vi "DIO 8-bit Bank.vi"(1 "DIO 7:0 Refnum":refnum<k21>, 2 "OUT 7:0":u8 format="%08b", 3 "DIR 7:0":u8 format="%08b") -> (0 "IN 7:0":u8 format="%08d")   [LabVIEW 2013]
uses:
  <vilib>/rvi/eio/common/nirviEmuTemplateMethod_errors.vi
  <vilib>/eio/EIOMethodNode/EIOMethodNode.xnode
  <vilib>/eio/EIONode/EIONode.xnode
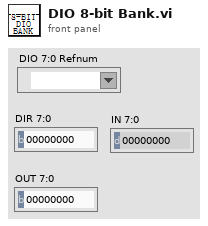
[diagram p1: front panel]
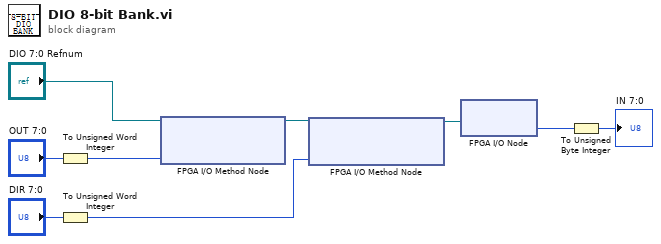
[diagram p0: block diagram]
diagram:
  n1 = To Unsigned Word Integer(number="OUT 7:0") -> (unsigned 16bit integer=w4:u16)
  n2 = To Unsigned Word Integer(number="DIR 7:0") -> (unsigned 16bit integer=w5:u16)
  n3 = xnode "FPGA I/O Method Node"("FPGA I/O In"="DIO 7:0 Refnum", "Data"=w4) -> ("FPGA I/O Out"=w1:refnum<k21>)
  n4 = xnode "FPGA I/O Method Node"("FPGA I/O In"=w1, "Enable"=w5) -> ("FPGA I/O Out"=w2:refnum<k21>)
  n5 = xnode "FPGA I/O Node"("FPGA I/O输入"=w2) -> ("I/O项"=w3:u16)  [unwired: 1 out]
  n6 = To Unsigned Byte Integer(number=w3) -> (unsigned 8bit integer=→"IN 7:0":u8)
